vi "ClusterReferernzenAufschluesseln.vi"(8 "error in (no error)":errorcluster caption="Fehler (Eingang, kein Fehler)", 11 "Cluster in":refnum<vi>[](array[refnum])) -> (0 "error out":errorcluster caption="Fehler (Ausgang)", 1 "Analysatoren":refnum<vi>[](array[refnum]), 2 "Ring Gasflasche aktiv out":refnum<vi>[](array[refnum]), 3 "Ring Components out":refnum<vi>[](array[refnum]))   [LabVIEW 2020, in "Linearisierung v2.lvlib" / "SpanEinstellungen.lvlib"]
uses:
  SpanEinstellungen.lvlib
  Seiten/System Einstellungen V2/System Einstellungen V2.lvlib
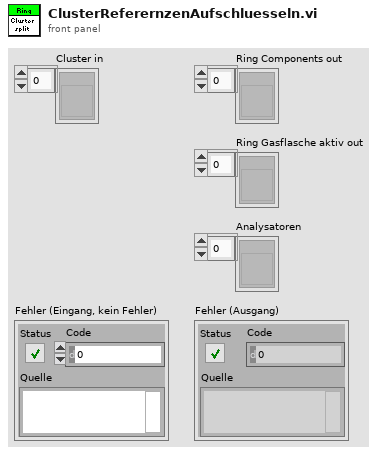
[diagram p1: front panel]
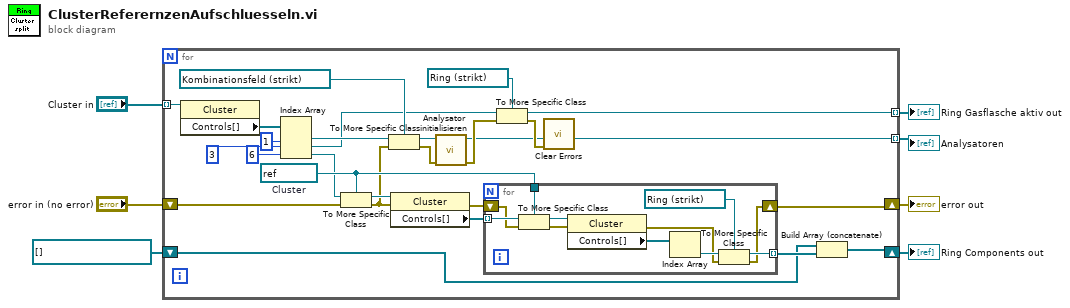
[diagram p0: block diagram]
diagram:
  n1 = for {
    tunnel: "Cluster in" -> [w31] mode=indexing
    shift-right: [w23] -> w7
    shift-left: refnum<vi>[] [] -> [w22]
    shift-right: [w17] -> w3
    shift-left: "error in (no error)" -> [w21]
    tunnel: [w13] -> w2 mode=indexing
    tunnel: [w8] -> w1 mode=indexing
    w25 = refnum<vi> refnum  # Cluster
    n2 = property class="Cluster"(reference=w31) -> ("Controls[]"=w33:refnum<vi>[])  [unwired: 1 in, 2 out]
    n3 = Index Array(array=w33, index #1=1 ("Index"), index #2=3 ("Index"), index #3=6 ("Index")) -> (element #1=w30:refnum<vi>, element #2=w14:refnum<vi>, element #3=w16:refnum<vi>)
    n4 = To More Specific Class(target class=w25, reference=w16, error in=w21) -> (specific class reference=w27:refnum<vi>, error out=w20:errorcluster)
    n5 = To More Specific Class(target class=refnum<vi> refnum ("Referenz Analysator"), reference=w30, error in=w20) -> (specific class reference=w28:refnum<vi>, error out=w19:errorcluster)
    n6 = property class="Cluster"(reference=w27, error in=w20) -> (error out=w18:errorcluster, "Controls[]"=w26:refnum<vi>[])  [unwired: 1 out]
    n7 = call "Analysator initialisieren.vi"("error in (no error)"=w19, "Referenz Analysator"=w28) -> ("error out"=w11:errorcluster, "Referenz Analysator out"=w8:refnum<vi>)  [unwired: 8 in]
    n8 = for {
      tunnel: w26 -> [w44] mode=indexing
      tunnel: w25 -> [w43]
      tunnel: [w39] -> w24 mode=indexing
      shift-right: [w34] -> w17
      shift-left: w18 -> [w37]
      n9 = To More Specific Class(target class=w43, reference=w44, error in=w37) -> (specific class reference=w42:refnum<vi>, error out=w36:errorcluster)
      n10 = property class="Cluster"(reference=w42, error in=w36) -> (error out=w35:errorcluster, "Controls[]"=w41:refnum<vi>[])  [unwired: 1 out]
      n11 = Index Array(array=w41) -> (element=w40:refnum<vi>)  [unwired: 1 in]
      n12 = To More Specific Class(target class=refnum<vi> refnum ("Komponente:"), reference=w40, error in=w35) -> (specific class reference=w39:refnum<vi>, error out=w34:errorcluster)
    }
    n13 = To More Specific Class(target class=refnum<vi> refnum ("Komponente:"), reference=w14, error in=w11) -> (specific class reference=w13:refnum<vi>, error out=w10:errorcluster)
    n14 = call <vilib>:"Clear Errors.vi"("error in (no error)"=w10) -> ()  [unwired: 5 in, 2 out]
    n15 = Build Array (concatenate)(w22, w24) -> (w23:refnum<vi>[])
  }
  "Ring Components out" <- w7
  "error out" <- w3
  "Ring Gasflasche aktiv out" <- w2
  "Analysatoren" <- w1
